vi "Variant to Class.vi"(8 "error in (no error)":errorcluster, 10 "Data in":variant, 11 "VIPB Build Node in":refnum<class "VIPB Build Node.lvclass">) -> (0 "error out":errorcluster, 2 "Data Out":variant, 3 "VIPB Build Node out":refnum<class "VIPB Build Node.lvclass">)   [LabVIEW 2014, in "VIPB Build Node.lvclass"]
uses:
  VIPB Build Node.lvclass
  Shared/Controls/VIPB Build - STYP.ctl
  VIPB Build Node.lvclass/VIPB Build Node.ctl
  Classes/Build Job/Build Job.lvclass
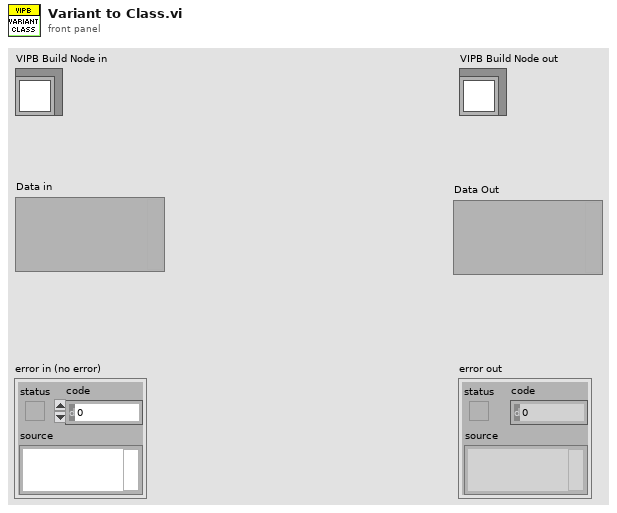
[diagram p1: front panel]
types:
  T1 = typedef "VIPB Build - STYP.ctl" = cluster{"VIPB Path":string, "Install after build":bool, "LabVIEW Version":string}
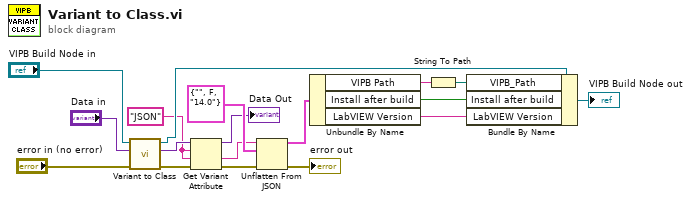
[diagram p0: block diagram]
diagram:
  w6 = "JSON" ("name")
  n1 = call-parent "Variant to Class.vi"("error in (no error)"="error in (no error)", "Data in"="Data in", "Build Job in"="VIPB Build Node in") -> ("error out"=w5:errorcluster, "Data Out"=w8:variant, "Build Job out"=w9:refnum<class "VIPB Build Node.lvclass">)  [unwired: 6 in]
  n2 = Get Variant Attribute(Variant=w8, name=w6, default value (empty Variant)=w6, error in=w5) -> (duplicate Variant=→"Data Out":variant, value=w11:string, error out=w10:errorcluster)  [unwired: 1 out]
  n3 = Unflatten From JSON(JSON string=w11, type and defaults=T1 {"VIPB Path"="", "Install after build"=FALSE, "LabVIEW Version"="14.0"} ("VIPB Build"), error in (no error)=w10) -> (value=w13:T1, error out=→"error out":errorcluster)  [unwired: 4 in]
  n4 = Unbundle By Name(w13) -> ("VIPB Path"=w14:string, "Install after build"=w2:bool, "LabVIEW Version"=w1:string)
  n5 = String To Path(string=w14) -> (path=w15:path)
  n6 = Bundle By Name(cluster=w9, "VIPB_Path"=w15, "Install after build"=w2, "LabVIEW Version"=w1) -> (→"VIPB Build Node out":refnum<class "VIPB Build Node.lvclass">)
